vi "unitsConversion.vi"(10 "Units":string) -> (2 "Numeric":dbl)   [LabVIEW 2014]
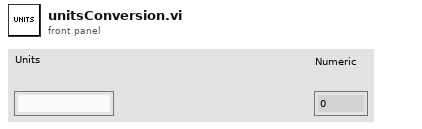
[diagram p1: front panel]
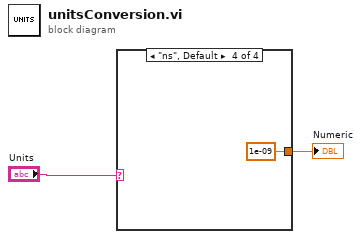
[diagram p0: block diagram]
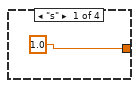
[diagram p2: hidden frame]
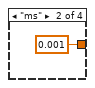
[diagram p3: hidden frame]
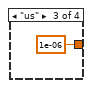
[diagram p4: hidden frame]
diagram:
  n1 = case shown="\"ns\", Default" "Units" {
    tunnel: [1.0 0.001 1e-06 1e-09] -> w1
    frame "s" {
    }
    frame "ms" {
    }
    frame "us" {
    }
    frame "ns", Default {
    }
  }
  "Numeric" <- w1
